vi "Test.vi"() -> ()   [LabVIEW 2020]
doc: "This VI is called when test mode begins, and will automatically be terminated when it ends. You can add manual or automatic tests and invoke them from the dashboard."
panel:
  in  "Default Tests":string[](array[string])=["Arm angle LEFT", "Arm angle RIGHT", "Climber LEFT", "Climber RIGHT", "ARM LEFT", "ARM RIGHT"]
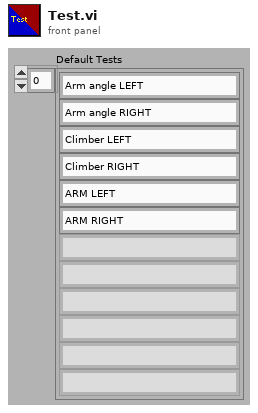
[diagram p1: front panel]
types:
  T1 = typedef "WPI_JoystickDevRef.ctl" = cluster{"Device":T2}
  T2 = typedef "WPI_JoystickDeviceEnum.ctl" = enum16{"USB 0", "USB 1", "USB 2", "USB 3", "USB 4", "USB 5"}
  T3 = typedef "WPI_MotorControlDeviceRef.ctl" = cluster{"DeviceStatus":errorcluster, "Type":T4, "PWM":cluster{"PWM Channel":T5, "DeadBand":T6}, "CAN":cluster{"Device Number":u8, "SetOutput VI Ref":variant, "GetOutput VI Ref":variant, "Enable VI Ref":variant, "Disable VI Ref":variant, "Data":variant}, "Invert":bool, "DIO PWM":cluster{"PWM \"Enable\" Channel":T5, "DIOChannel":T7, "PWM Rate":dbl}}
  T4 = typedef "WPI_MotorControlType.ctl" = enum16{"PWM", "CAN", "DIO PWM"}
  T5 = typedef "FPGA_DIOPWMChannel.ctl" = enum8{"PWM 0", "PWM 1", "PWM 2", "PWM 3", "PWM 4", "PWM 5", "PWM 6", "PWM 7", "PWM 8", "PWM 9", "PWM MXP 0", "PWM MXP 1", "PWM MXP 2", "PWM MXP 3", "PWM MXP 4", "PWM MXP 5", "PWM MXP 6", "PWM MXP 7", "PWM MXP 8", "PWM MXP 9", "Invalid"}
  T6 = typedef "WPI_PWMDeadband.ctl" = cluster{"Name":string, "maxPositivePwm":i32, "minPositivePwm":i32, "centerPwm":i32, "maxNegativePwm":i32, "minNegativePwm":i32, "angularRange":u16}
  T7 = typedef "FPGA_DIOChannel.ctl" = enum8{"DIO 0", "DIO 1", "DIO 2", "DIO 3", "DIO 4", "DIO 5", "DIO 6", "DIO 7", "DIO 8", "DIO 9", "DIO MXP 0", "DIO MXP 1", "DIO MXP 2", "DIO MXP 3", "DIO MXP 4", "DIO MXP 5", "DIO MXP 6", "DIO MXP 7", "DIO MXP 8", "DIO MXP 9", "DIO MXP 10", "DIO MXP 11", "DIO MXP 12", "DIO MXP 13", "DIO MXP 14", "DIO MXP 15", "SPI Port CS1", "SPI Port CS2", "SPI Port CS3", "SPI Port MISO", "SPI Port MOSI", "Invalid"}
  T8 = cluster{"JoystickDevRef":T1, "PhoenixMotorControlDevRef":T3}
  T9 = cluster{"JoystickDevRef":T1, "MotorControlDevRef":T3}
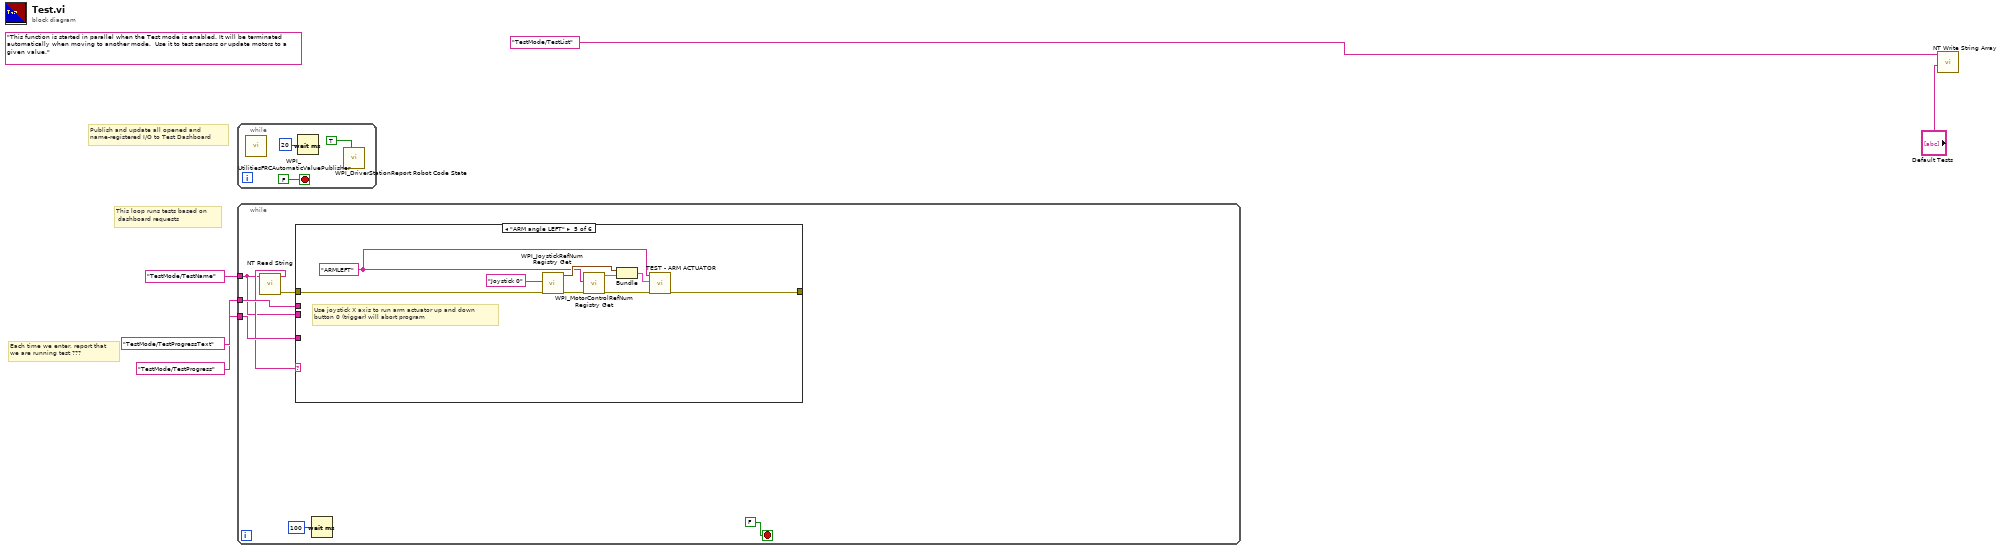
[diagram p0: block diagram]
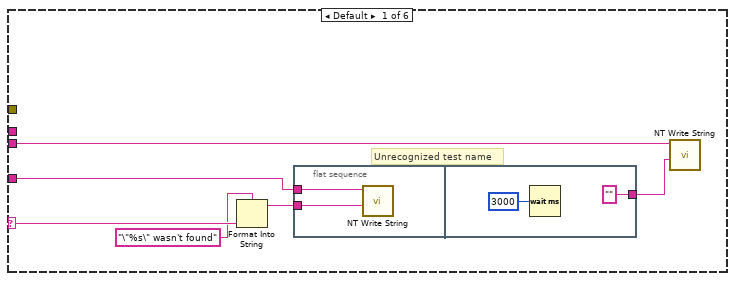
[diagram p2: hidden frame]
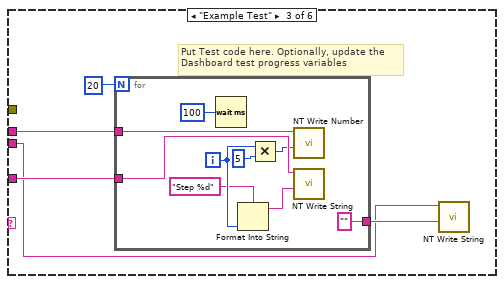
[diagram p4: hidden frame]
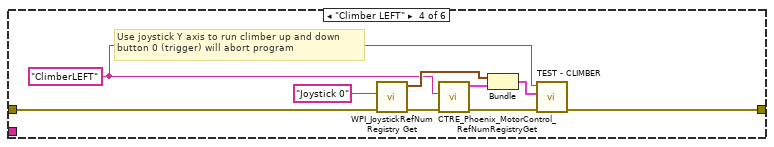
[diagram p5: hidden frame]
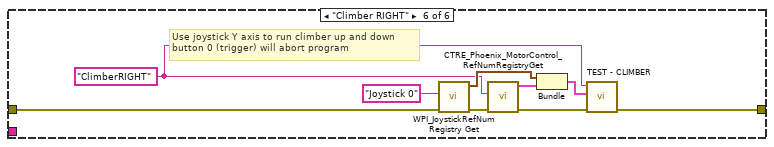
[diagram p6: hidden frame]
diagram:
  (unwired) "This function is started in parallel when the Test mode is enabled. It will be terminated automatically when moving to another mode.  Use it to test sensors or update motors to a given value."
  # "This loop runs tests based on \n dashboard requests"
  # "Publish and update all opened and\nname-registered I/O to Test Dashboard"
  # "Each time we enter, report that\nwe are running test ???"
  n1 = while {
    stop <- FALSE stop-if-true
    n2 = call <vilib>:"WPI_UtilitiesFRCAutomaticValuePublisher.vi"() -> ()  [unwired: 12 in]
    n3 = Wait (ms)(milliseconds to wait=u32 20) -> ()  [unwired: 1 out]
    n4 = call <vilib>:"WPI_DriverStationReport Robot Code State.vi"("Test"=TRUE ("Autonomous")) -> ()  [unwired: 10 in, 1 out]
  }
  n5 = while {
    tunnel: "TestMode/TestName" ("Name") -> [w10]
    tunnel: "TestMode/TestProgressText" ("Name") -> [w13]
    tunnel: "TestMode/TestProgress" ("Name") -> [w12]
    stop <- FALSE stop-if-true
    n6 = call <vilib>:"NT Read String.vi"("Name"=w10) -> ("error out"=w9:errorcluster, "String"=w11:string)  [unwired: 9 in]
    n7 = case shown="\"ARM angle LEFT\"" w11 {
      selector: w11 -> [w20 _ _ _ _ _]
      tunnel: w10 -> [w17 _ w26 _ _ _]
      tunnel: w13 -> [w21 _ w29 _ _ _]
      tunnel: w12 -> [_ _ w30 _ _ _]
      tunnel: w9 -> [_ _ _ w42 w53 w60]
      tunnel: [_ _ _ w40 w52 w58] -> _
      frame Default {
        # "Unrecognized test name"
        n8 = Format Into String(format string="\"%s\" wasn't found" ("Name"), w20) -> (resulting string=w19:string)  [unwired: 2 in, 1 out]
        n9 = flat-sequence {
          tunnel: w21 -> [w22]
          tunnel: w19 -> [w23]
          tunnel: ["" ("Name")] -> w16
          frame #0 {
            n10 = call <vilib>:"NT Write String.vi"("String"=w23, "Name"=w22) -> ()  [unwired: 9 in, 1 out]
          }
          frame #1 {
            n11 = Wait (ms)(milliseconds to wait=u32 3000) -> ()  [unwired: 1 out]
          }
        }
        n12 = call <vilib>:"NT Write String.vi"("String"=w16, "Name"=w17) -> ()  [unwired: 9 in, 1 out]
      }
      frame "" {
        # "No test to run"
      }
      frame "Example Test" {
        # "Put Test code here. Optionally, update the\nDashboard test progress variables"
        n13 = for {
          N: 20 -> [_]
          tunnel: w30 -> [w39]
          tunnel: w29 -> [w37]
          tunnel: ["" ("String")] -> w27
          i -> [w34]
          n14 = Wait (ms)(milliseconds to wait=u32 100) -> ()  [unwired: 1 out]
          n15 = Format Into String(format string="Step %d", w34) -> (resulting string=w32:string)  [unwired: 2 in, 1 out]
          n16 = Multiply(x=w34, y=u32 5 ("milliseconds to wait")) -> (x*y=w35:u32)
          n17 = call <vilib>:"NT Write Number.vi"("Numeric"=w35, "Name"=w39) -> ()  [unwired: 9 in, 1 out]
          n18 = call <vilib>:"NT Write String.vi"("String"=w32, "Name"=w37) -> ()  [unwired: 9 in, 1 out]
        }
        n19 = call <vilib>:"NT Write String.vi"("String"=w27, "Name"=w26) -> ()  [unwired: 9 in, 1 out]
      }
      frame "Climber LEFT" {
        w43 = "ClimberLEFT" ("refnum name")
        # "Use joystick Y axis to run climber up and down\nbutton 0 (trigger) will abort program"
        n20 = call <vilib>:"WPI_JoystickRefNum Registry Get.vi"("error in (no error)"=w42, "refnum name"="Joystick 0") -> ("error out"=w44:errorcluster, "JoystickDevRef"=w47:T1)  [unwired: 8 in]
        n21 = call <vilib>:"CTRE_Phoenix_MotorControl_RefNumRegistryGet.vi"("error in (no error)"=w44, "refnum name"=w43) -> ("error out"=w41:errorcluster, "PhoenixMotorControlDevRef"=w46:T3)  [unwired: 8 in]
        n22 = Bundle("JoystickDevRef"=w47, "PhoenixMotorControlDevRef"=w46) -> (w45:T8)  [unwired: 1 in]
        n23 = call "TEST - CLIMBER.vi"("error in (no error)"=w41, "Cluster of JOYSTICK and CLIMBER ref info"=w45, "refnum name"=w43) -> ("error out"=w40:errorcluster)  [unwired: 8 in]
      }
      frame "ARM angle LEFT" {
        w49 = "ARMLEFT" ("refnum name")
        # "Use joystick X axis to run arm actuator up and down\nbutton 0 (trigger) will abort program"
        n24 = call <vilib>:"WPI_JoystickRefNum Registry Get.vi"("error in (no error)"=w53, "refnum name"="Joystick 0") -> ("error out"=w54:errorcluster, "JoystickDevRef"=w56:T1)  [unwired: 8 in]
        n25 = call <vilib>:"WPI_MotorControlRefNum Registry Get.vi"("error in (no error)"=w54, "refnum name"=w49) -> ("error out"=w51:errorcluster, "MotorControlDevRef"=w55:T3)  [unwired: 8 in]
        n26 = Bundle("JoystickDevRef"=w56, "MotorControlDevRef"=w55) -> (w50:T9)  [unwired: 1 in]
        n27 = call "TEST - ARM ACTUATOR.vi"("error in (no error)"=w51, "Cluster of JOYSTICK and ARM ACTUATOR ref info"=w50, "refnum name"=w49) -> ("error out"=w52:errorcluster)  [unwired: 8 in]
      }
      frame "Climber RIGHT" {
        w61 = "ClimberRIGHT" ("refnum name")
        # "Use joystick Y axis to run climber up and down\nbutton 0 (trigger) will abort program"
        n28 = call <vilib>:"WPI_JoystickRefNum Registry Get.vi"("error in (no error)"=w60, "refnum name"="Joystick 0") -> ("error out"=w62:errorcluster, "JoystickDevRef"=w65:T1)  [unwired: 8 in]
        n29 = call <vilib>:"CTRE_Phoenix_MotorControl_RefNumRegistryGet.vi"("error in (no error)"=w62, "refnum name"=w61) -> ("error out"=w59:errorcluster, "PhoenixMotorControlDevRef"=w64:T3)  [unwired: 8 in]
        n30 = Bundle("JoystickDevRef"=w65, "PhoenixMotorControlDevRef"=w64) -> (w63:T8)  [unwired: 1 in]
        n31 = call "TEST - CLIMBER.vi"("error in (no error)"=w59, "Cluster of JOYSTICK and CLIMBER ref info"=w63, "refnum name"=w61) -> ("error out"=w58:errorcluster)  [unwired: 8 in]
      }
    }
    n32 = Wait (ms)(milliseconds to wait=u32 100) -> ()  [unwired: 1 out]
  }
  n33 = call <vilib>:"NT Write String Array.vi"("String Array"="Default Tests", "Name"="TestMode/TestList") -> ()  [unwired: 9 in, 1 out]
